vi "Global 3.vi"() -> ()   [LabVIEW 2016]
panel:
  out "Имя":string
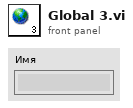
[diagram p1: front panel]
diagram:
